vi "Create Measurement Service.vi"() -> ()   [LabVIEW 2020, in "MeasurementService Editor.lvlib"]
uses:
  _Editor/MeasurementService Editor.lvlib
  <vilib>/Utility/error.llb/ErrWarn.ctl
panel:
  in  "Measurement Plug-in Description":string
  out "Status":T1=TRUE caption="Measurement plug-in name must be unique and cannot contain any of the following characters:\n           \\ / : * ? \" < > |"
  in  "Create Measurement Service":bool
  in  "Measurement Plug-in Name":string
  out "Active Project Name":string
  # "* Project in which the measurement plug-in will be created"
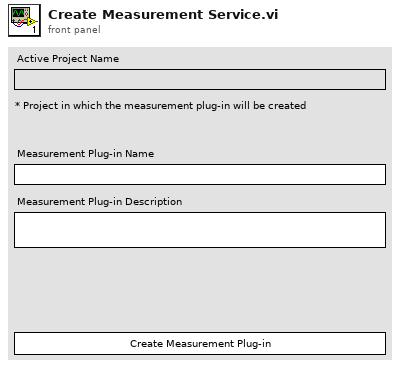
[diagram p1: front panel]
types:
  T1 = typedef "ErrWarn.ctl" = bool
  T2 = enum8{"Enabled", "Disabled", "Disabled and Grayed Out"}
  T3 = cluster{"project ref":refnum<vi>, "measurement plug-in name":string, "measurement plug-in description":string}
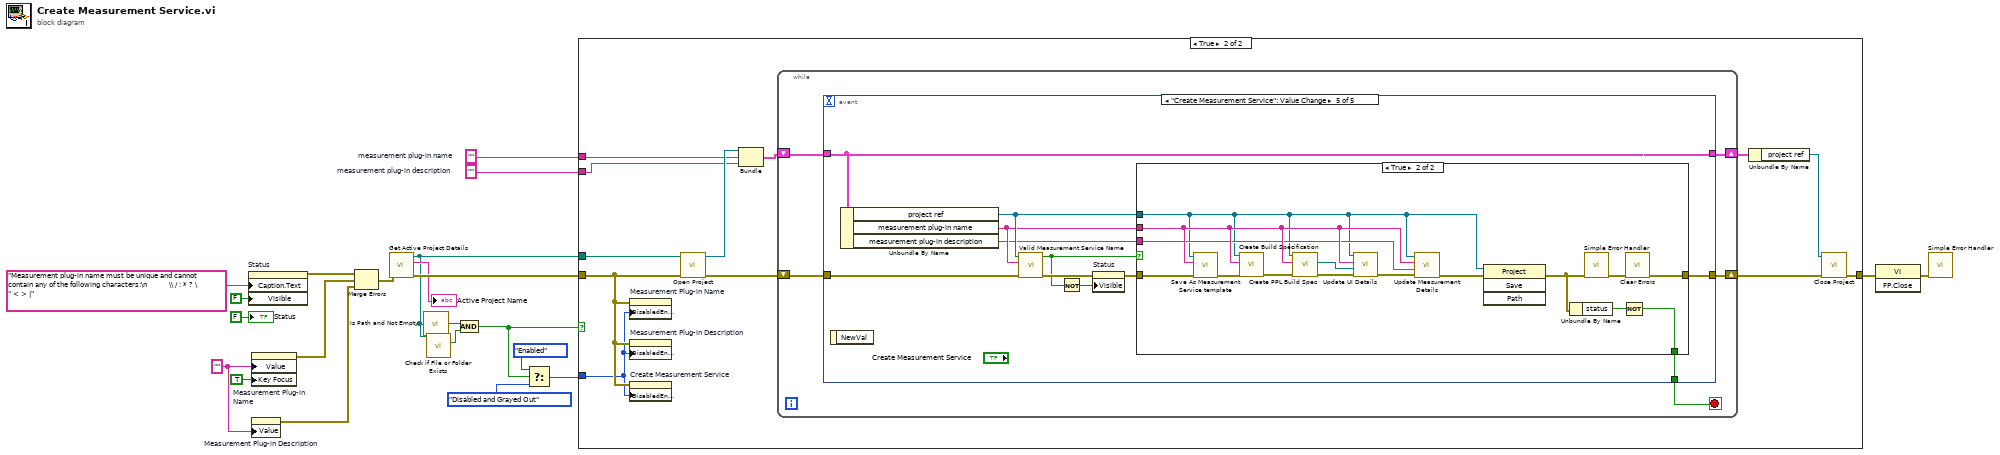
[diagram p0: block diagram]
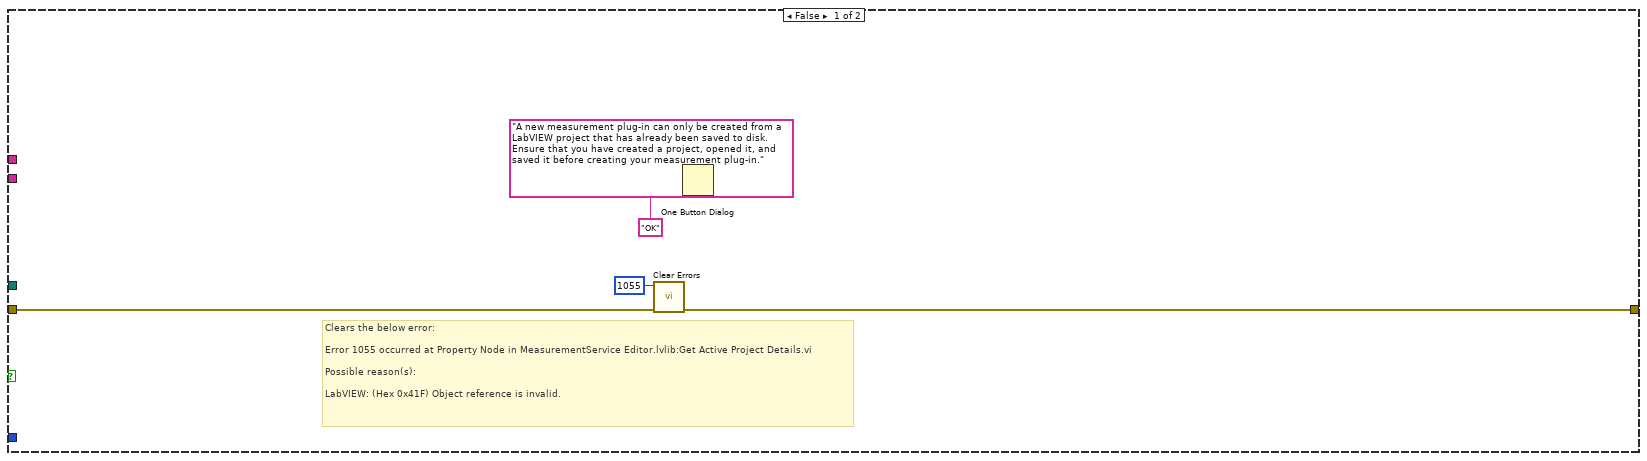
[diagram p2: hidden frame]
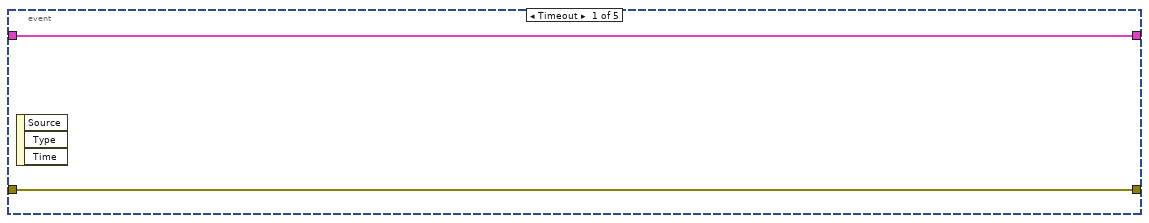
[diagram p3: hidden frame]
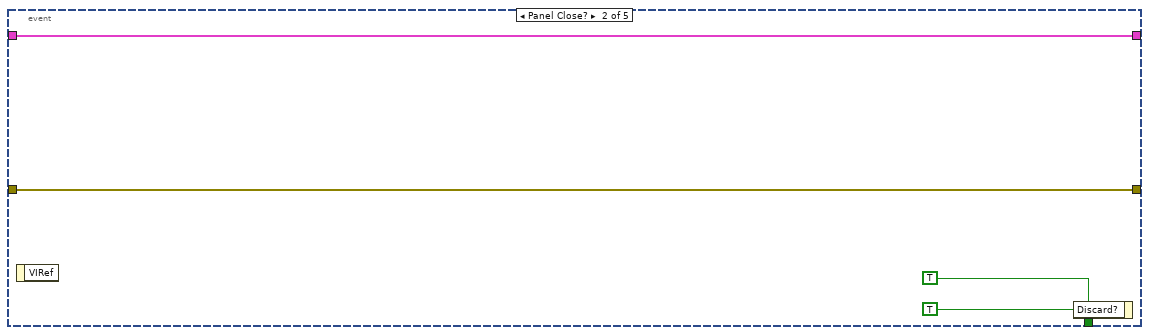
[diagram p4: hidden frame]
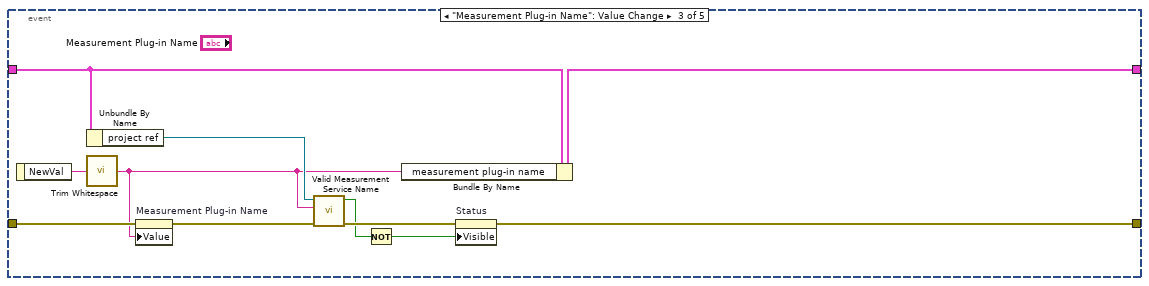
[diagram p5: hidden frame]
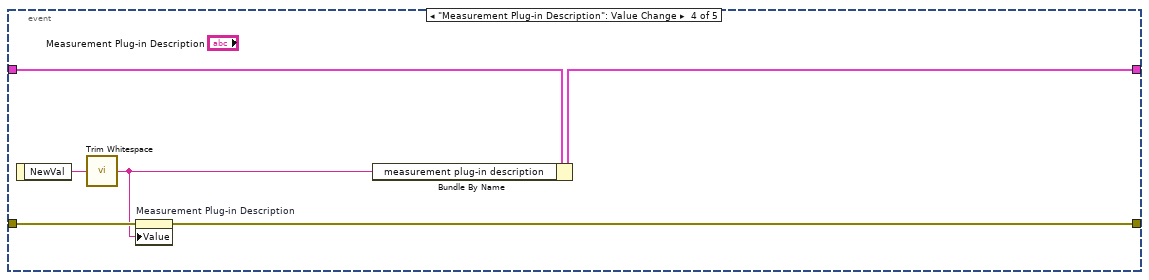
[diagram p6: hidden frame]
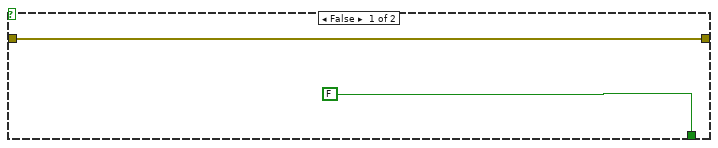
[diagram p7: hidden frame]
diagram:
  w3 = ""  # measurement plug-in description
  w2 = "" ("Measurement Service Name")
  w22 = ""  # measurement plug-in name
  n1 = property on="Status" class="Bool"("Caption.Text"="Measurement plug-in name must be unique and cannot contain any of the following characters:\n           \\ / : * ? \" < > |" ("Status"), "Visible"=FALSE) -> (error out=w19:errorcluster)  [unwired: 2 in, 1 out]
  n2 = property on="Measurement Plug-in Name" class="Str"("Value"=w2, "Key Focus"=TRUE) -> (error out=w17:errorcluster)  [unwired: 2 in, 1 out]
  n3 = property on="Measurement Plug-in Description" class="Str"("Value"=w2) -> (error out=w1:errorcluster)  [unwired: 2 in, 1 out]
  n4 = Merge Errors(w19, w17, w1) -> (w18:errorcluster)
  n5 = call "Get Active Project Details.vi"("error in"=w18) -> ("error out"=w14:errorcluster, "name"=→"Active Project Name":string, "path"=w9:path)  [unwired: 8 in]
  n6 = call <vilib>:"Is Path and Not Empty.vi"("path"=w9) -> ("Is Path and Not Empty?"=w8:bool)  [unwired: 4 in]
  n7 = call <vilib>:"Check if File or Folder Exists.vi"("path"=w9) -> ("file or folder exists?"=w7:bool)  [unwired: 8 in, 2 out]
  n8 = And(x=w8, y=w7) -> (x .and. y?=w6:bool)
  n9 = Select(t=T2."Enabled" ("Disabled"), s=w6, f=T2."Disabled and Grayed Out" ("Disabled")) -> (s? t:f=w10:T2)
  n10 = case shown="True" w6 {
    tunnel: w22 -> [_ w33]
    tunnel: [w24 w32] -> w16
    tunnel: w14 -> [w27 w29]
    tunnel: w10 -> [_ w28]
    tunnel: w9 -> [_ w31]
    tunnel: w3 -> [_ w30]
    frame False {
      # "Clears the below error:\n\nError 1055 occurred at Property Node in MeasurementService Editor.lvlib:Get Active Project Details.vi\n\nPossible reason(s):\n\nLabVIEW: (Hex 0x41F) Object reference is invalid."
      n11 = call <vilib>:"Clear Errors.vi"("error in (no error)"=w27, "specific error code to clear (0: all)"=1055) -> ("error out"=w24:errorcluster)  [unwired: 4 in, 1 out]
      n12 = One Button Dialog(message="A new measurement plug-in can only be created from a LabVIEW project that has already been saved to disk.  Ensure that you have created a project, opened it, and saved it before creating your measurement plug-in.", button name ("OK")="OK") -> ()  [unwired: 1 out]
    }
    frame True {
      n13 = property on="Measurement Plug-in Name" class="Str"(error in=w29, "DisabledEnum"=w28) -> ()  [unwired: 1 in, 2 out]
      n14 = property on="Measurement Plug-in Description" class="Str"(error in=w29, "DisabledEnum"=w28) -> ()  [unwired: 1 in, 2 out]
      n15 = property on="Create Measurement Service" class="Bool"(error in=w29, "DisabledEnum"=w28) -> ()  [unwired: 1 in, 2 out]
      n16 = call "Open Project.vi"("error in"=w29, "path"=w31) -> ("error out"=w39:errorcluster, "project ref"=w38:refnum<vi>)  [unwired: 8 in]
      n17 = Bundle("project ref"=w38, "measurement plug-in name"=w33, "measurement plug-in description"=w30) -> (w37:T3)  [unwired: 1 in]
      n18 = while {
        shift-right: [w43] -> w34
        shift-left: w39 -> [w42]
        shift-right: [w40] -> w36
        shift-left: w37 -> [w41]
        stop <- w44 stop-if-true
        n19 = event shown="[4] \"Create Measurement Service\": Value Change" {
          selector: _ -> [_ _ _ _ _]
          dyn-events: _ -> [_ _ _ _ _]
          timeout: _ -> [_ _ _ _ _]
          tunnel: [_ TRUE ("Discard?") _ _ w71] -> w44
          tunnel: [w46 w48 w57 w63 w72] -> w43
          tunnel: w42 -> [w46 w48 w53 w64 w77]
          tunnel: w41 -> [w45 w47 w56 w66 w78]
          tunnel: [w45 w47 w61 w65 w78] -> w40
          event Timeout {
            n20 = event-data() -> ()  [unwired: 1 in, 3 out]
          }
          event Panel Close? {
            n21 = event-data() -> ()  [unwired: 1 in, 1 out]
            n22 = event-data("Discard?"=TRUE) -> ()  [unwired: 1 in, 1 out]
          }
          event "Measurement Plug-in Name": Value Change {
            n23 = event-data() -> ("NewVal"=w54:string)  [unwired: 1 in]
            n24 = Unbundle By Name(w56) -> ("project ref"=w55:refnum<vi>)
            n25 = call <vilib>:"Trim Whitespace.vi"("string"=w54) -> ("trimmed string"=w51:string)  [unwired: 1 in]
            n26 = property on="Measurement Plug-in Name" class="Str"(error in=w53, "Value"=w51) -> (error out=w52:errorcluster)  [unwired: 1 in, 1 out]
            n27 = call "Valid Measurement Service Name.vi"("error in"=w52, "requested plugin name"=w51, "project ref"=w55) -> ("error out"=w60:errorcluster, "valid name?"=w58:bool)  [unwired: 7 in]
            n28 = Not(x=w58) -> (.not. x?=w59:bool)
            n29 = Bundle By Name(cluster=w56, "measurement plug-in name"=w51) -> (w61:T3)
            n30 = property on="Status" class="Bool"(error in=w60, "Visible"=w59) -> (error out=w57:errorcluster)  [unwired: 1 in, 1 out]
          }
          event "Measurement Plug-in Description": Value Change {
            n31 = event-data() -> ("NewVal"=w67:string)  [unwired: 1 in]
            n32 = call <vilib>:"Trim Whitespace.vi"("string"=w67) -> ("trimmed string"=w62:string)  [unwired: 1 in]
            n33 = property on="Measurement Plug-in Description" class="Str"(error in=w64, "Value"=w62) -> (error out=w63:errorcluster)  [unwired: 1 in, 1 out]
            n34 = Bundle By Name(cluster=w66, "measurement plug-in description"=w62) -> (w65:T3)
          }
          event "Create Measurement Service": Value Change {
            n35 = event-data() -> ()  [unwired: 1 in, 1 out]
            n36 = Unbundle By Name(w78) -> ("project ref"=w70:refnum<vi>, "measurement plug-in name"=w69:string, "measurement plug-in description"=w68:string)
            n37 = call "Valid Measurement Service Name.vi"("error in"=w77, "requested plugin name"=w69, "project ref"=w70) -> ("error out"=w76:errorcluster, "valid name?"=w74:bool)  [unwired: 7 in]
            n38 = Not(x=w74) -> (.not. x?=w75:bool)
            n39 = property on="Status" class="Bool"(error in=w76, "Visible"=w75) -> (error out=w73:errorcluster)  [unwired: 1 in, 1 out]
            n40 = case shown="True" w74 {
              tunnel: w73 -> [w80 w95]
              tunnel: [w80 w91] -> w72
              tunnel: [FALSE w93] -> w71
              tunnel: w70 -> [_ w86]
              tunnel: w69 -> [_ w88]
              tunnel: w68 -> [_ w87]
              frame False {
              }
              frame True {
                n41 = call "Save As Measurement Service template.vi"("error in"=w95, "measurement service name"=w88, "project ref"=w86) -> ("error out"=w81:errorcluster)  [unwired: 8 in]
                n42 = call "Create Build Specification.vi"("error in"=w81, "measurement service name"=w88, "project in"=w86) -> ("error out"=w85:errorcluster)  [unwired: 8 in]
                n43 = call "Create PPL Build Spec.vi"("error in (no error)"=w85, "measurement plug-in name"=w88, "project refnum"=w86) -> ("error out"=w84:errorcluster, "measurement UI built path"=w82:path)  [unwired: 7 in]
                n44 = call "Update UI Details.vi"("error in"=w84, "UI path"=w82, "measurement service name"=w88, "project ref"=w86) -> ("error out"=w83:errorcluster)  [unwired: 7 in]
                n45 = call "Update Measurement Details.vi"("error in"=w83, "measurement service description"=w87, "measurement service name"=w88, "project ref"=w86) -> ("error out"=w90:errorcluster)  [unwired: 7 in]
                n46 = invoke class="Project" method="Save"(reference=w86, error in=w90) -> (error out=w89:errorcluster)  [unwired: 2 in, 3 out]
                n47 = Unbundle By Name(w89) -> ("status"=w94:bool)
                n48 = call <vilib>:"Simple Error Handler.vi"("error in (no error)"=w89) -> ("error out"=w92:errorcluster)  [unwired: 4 in, 4 out]
                n49 = Not(x=w94) -> (.not. x?=w93:bool)
                n50 = call <vilib>:"Clear Errors.vi"("error in (no error)"=w92) -> ("error out"=w91:errorcluster)  [unwired: 5 in, 1 out]
              }
            }
          }
        }
      }
      n51 = Unbundle By Name(w36) -> ("project ref"=w35:refnum<vi>)
      n52 = call "Close Project.vi"("error in"=w34, "project ref"=w35) -> ("error out"=w32:errorcluster)  [unwired: 9 in]
    }
  }
  n53 = invoke class="VI" method="FP.Close"(error in=w16) -> (error out=w15:errorcluster)  [unwired: 2 in, 2 out]
  n54 = call <vilib>:"Simple Error Handler.vi"("error in (no error)"=w15) -> ()  [unwired: 4 in, 5 out]
  "Status" <- T1 FALSE ("Status")
